vi "Aim.vi"(1 "Aim":bool) -> (0 "Ready":bool)   [LabVIEW 2013]
uses:
  Robot Global Data.vi
panel:
  in  "Aim Position":dbl=75.0
  in  "Open Position":dbl=115.0
  in  "Closed Position":dbl
  in  "Rest Speed r/s":dbl=15.0 min=0.0 max=0.7 step=0.05
  # "15"
  # "0"
  # "Gate Servo"
  # "60"
  # "90"
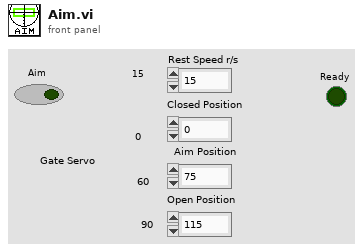
[diagram p1: front panel]
types:
  T1 = typedef "WPI_ServoDeviceRef.ctl" = cluster{"DeviceStatus":errorcluster, "Digital Module":T2, "PWM Channel":T3, "DeadBand":T4}
  T2 = typedef "FPGA_TypedefDigitalModule.ctl" = enum16{"Digital Module 1", "Digital Module 2"}
  T3 = typedef "FPGA_DIOPWMChannel.ctl" = enum8{"PWM 1", "PWM 2", "PWM 3", "PWM 4", "PWM 5", "PWM 6", "PWM 7", "PWM 8", "PWM 9", "PWM 10", "Invalid"}
  T4 = typedef "WPI_PWMDeadband.ctl" = cluster{"Name":string, "maxPositivePwm":i32, "minPositivePwm":i32, "centerPwm":i32, "maxNegativePwm":i32, "minNegativePwm":i32, "angularRange":u16}
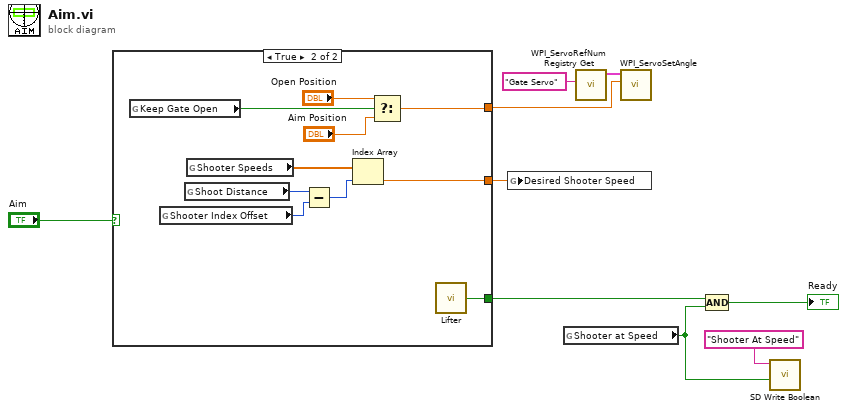
[diagram p0: block diagram]
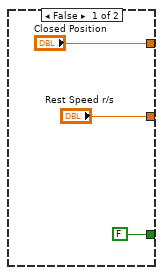
[diagram p2: hidden frame]
diagram:
  n1 = case shown="True" "Aim" {
    tunnel: ["Closed Position" w22] -> w7
    tunnel: [FALSE w18] -> w3
    tunnel: ["Rest Speed r/s" w13] -> w5
    frame False {
    }
    frame True {
      n2 = global read "Robot Global Data.vi" "Keep Gate Open"() -> (w19:bool)
      n3 = global read "Robot Global Data.vi" "Shooter Index Offset"() -> (w16:i32)
      n4 = global read "Robot Global Data.vi" "Shoot Distance"() -> (w14:i32)
      n5 = global read "Robot Global Data.vi" "Shooter Speeds"() -> (w17:dbl[])
      n6 = Subtract(x=w14, y=w16) -> (x-y=w15:i32)
      n7 = Index Array(array=w17, index=w15) -> (element=w13:dbl)
      n8 = Select(t="Open Position", s=w19, f="Aim Position") -> (s? t:f=w22:dbl)
      n9 = call "Lifter.vi"() -> ("In Position"=w18:bool)  [unwired: 1 in]
    }
  }
  n10 = global write "Robot Global Data.vi" "Desired Shooter Speed"(w5) -> ()
  n11 = global read "Robot Global Data.vi" "Shooter at Speed"() -> (w1:bool)
  n12 = call <vilib>:"WPI_ServoRefNum Registry Get.vi"("refnum name"="Gate Servo") -> ("ServoDeviceRef"=w9:T1)  [unwired: 9 in, 1 out]
  n13 = call <vilib>:"WPI_ServoSetAngle.vi"("Angle"=w7, "ServoDeviceRef"=w9) -> ()  [unwired: 8 in, 2 out]
  n14 = Compound Arithmetic op=AND(w3, w1) -> (→"Ready":bool)
  n15 = call <vilib>:"SD Write Boolean.vi"("Boolean"=w1, "Name"="Shooter At Speed") -> ()  [unwired: 8 in, 2 out]
